vi "sendCenterTarget.vi"(11 "Target Info":T1(array[cluster])) -> ()   [LabVIEW 2012]
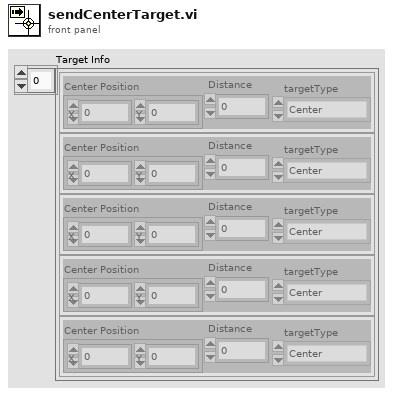
[diagram p1: front panel]
types:
  T1 = cluster{"Center Position":cluster{"X":dbl, "Y":dbl}, "Distance":dbl, "targetType":enum16{"Center", "Side", "Vertical"}}[]
  T2 = enum16{"Invalid", "Center", "TwoSides", "TwoVerticals", "SideAndVert", "OneSide"}
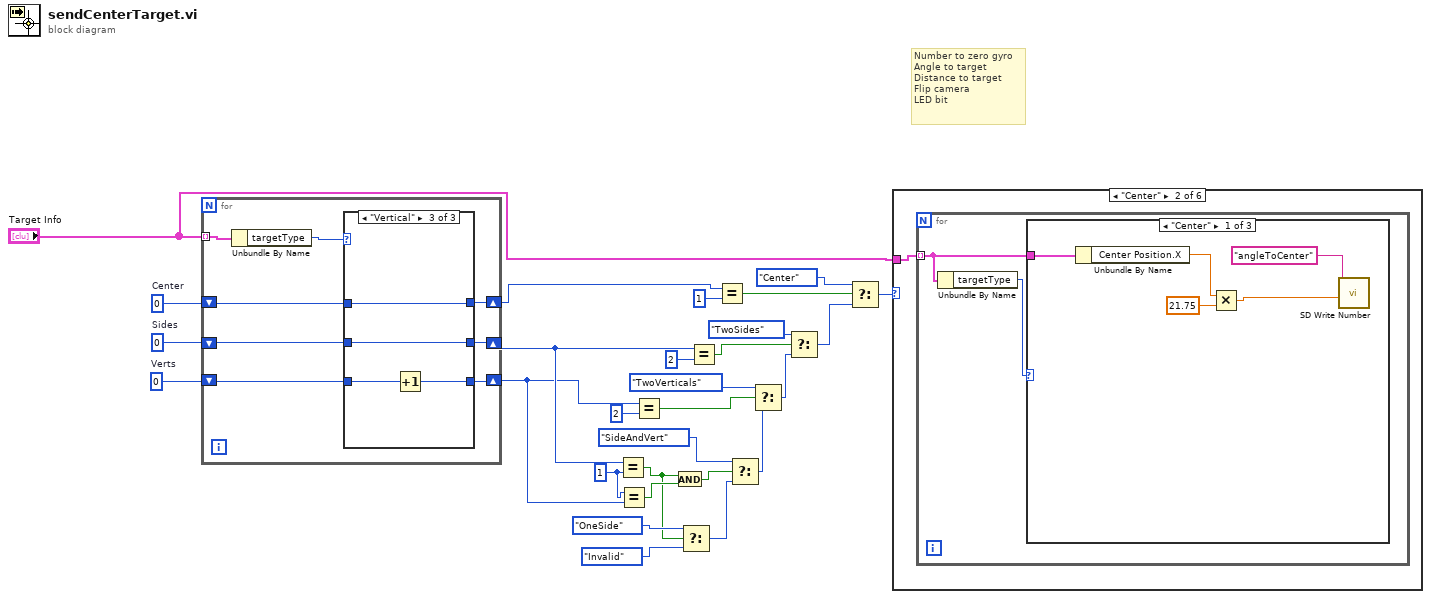
[diagram p0: block diagram]
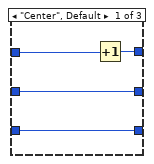
[diagram p9: hidden frame]
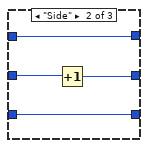
[diagram p10: hidden frame]
diagram:
  w8 = 1 ("y")
  w26 = 0  # Verts
  w27 = 0  # Sides
  w28 = 0  # Center
  # "Number to zero gyro\nAngle to target\nDistance to target\nFlip camera\nLED bit"
  n1 = for {
    tunnel: "Target Info" -> [w36] mode=indexing
    shift-right: [w33] -> w18
    shift-left: w28 -> [w34]
    shift-right: [w32] -> w10
    shift-left: w27 -> [w31]
    shift-right: [w30] -> w9
    shift-left: w26 -> [w29]
    n2 = Unbundle By Name(w36) -> ("targetType"=w35:enum16{"Center", "Side", "Vertical"})
    n3 = case shown="\"Vertical\"" w35 {
      tunnel: w34 -> [w40 w42 w46]
      tunnel: [w39 w42 w46] -> w33
      tunnel: [w38 w43 w45] -> w32
      tunnel: w31 -> [w38 w44 w45]
      tunnel: [w37 w41 w47] -> w30
      tunnel: w29 -> [w37 w41 w48]
      frame "Center", Default {
        n4 = Increment(x=w40) -> (x+1=w39:i32)
      }
      frame "Side" {
        n5 = Increment(x=w44) -> (x+1=w43:i32)
      }
      frame "Vertical" {
        n6 = Increment(x=w48) -> (x+1=w47:i32)
      }
    }
  }
  n7 = Equal?(x=w10, y=w8) -> (x = y?=w3:bool)
  n8 = Equal?(x=w8, y=w9) -> (x = y?=w7:bool)
  n9 = Equal?(x=w9, y=2) -> (x = y?=w14:bool)
  n10 = And(x=w3, y=w7) -> (x .and. y?=w6:bool)
  n11 = Select(t=T2."OneSide" ("y"), s=w3, f=T2."Invalid" ("y")) -> (s? t:f=w5:T2)
  n12 = Equal?(x=w10, y=2) -> (x = y?=w16:bool)
  n13 = Equal?(x=w18, y=1) -> (x = y?=w19:bool)
  n14 = Select(t=T2."SideAndVert" ("y"), s=w6, f=w5) -> (s? t:f=w12:T2)
  n15 = Select(t=T2."TwoVerticals" ("y"), s=w14, f=w12) -> (s? t:f=w15:T2)
  n16 = Select(t=T2."TwoSides" ("y"), s=w16, f=w15) -> (s? t:f=w21:T2)
  n17 = Select(t=T2."Center" ("y"), s=w19, f=w21) -> (s? t:f=w23:T2)
  n18 = case shown="\"Center\"" w23 {
    tunnel: "Target Info" -> [_ w49 _ _ _ _]
    frame "Invalid", Default {
    }
    frame "Center" {
      n19 = for {
        tunnel: w49 -> [w51] mode=indexing
        n20 = Unbundle By Name(w51) -> ("targetType"=w50:enum16{"Center", "Side", "Vertical"})
        n21 = case shown="\"Center\"" w50 {
          tunnel: w51 -> [w52 _ _]
          frame "Center" {
            n22 = Unbundle By Name(w52) -> ("Center Position.X"=w53:dbl)
            n23 = Multiply(x=w53, y=21.75) -> (x*y=w54:dbl)
            n24 = call <vilib>:"SD Write Number.vi"("Numeric"=w54, "Name"="angleToCenter") -> ()  [unwired: 8 in, 2 out]
          }
          frame "Side" {
          }
          frame "Vertical" {
          }
        }
      }
    }
    frame "TwoSides" {
    }
    frame "TwoVerticals" {
    }
    frame "SideAndVert" {
    }
    frame "OneSide" {
    }
  }
